vi "Apply Module Configuration Data.vi"(8 "Error In":errorcluster, 11 "Compiled.Settings":T1 {"Configuration Data"."Properties"."U64 Properties"."UInt64 Write" format="%.0x"; "Configuration Data"."Properties"."U32 Properties"."UInt32 Write" format="%.0x"; "Configuration Data"."Properties"."Double Properties"."Double Write" format="%_20g"}) -> (0 "Error Out":errorcluster, 2 "Device Session":refnum<k21>, 3 "SLSC Module Name":refnum<k21>)   [LabVIEW 2015, in "SLSC-12201 DIO Engine.lvlib"]
uses:
  SLSC-12201 DIO Engine.lvlib
  Shared/Compiled.Settings
  Shared/SLSC Dynamic Channel.ctl
  Shared/SLSC Dynamic Channel Type.ctl
  <vilib>/SLSC/Initialize Session with Devices.vi
  <vilib>/NI Veristand/Custom Device Tools/Custom Device Utility Library/Custom Device Utility Library.lvlib
  <vilib>/NI Veristand/Custom Device Tools/Custom Device Utility Library/RT Debug String Color Spec.ctl
  <vilib>/SLSC/SLSC.lvlib
  Shared/SLSC-12201 DIO Shared.lvlib
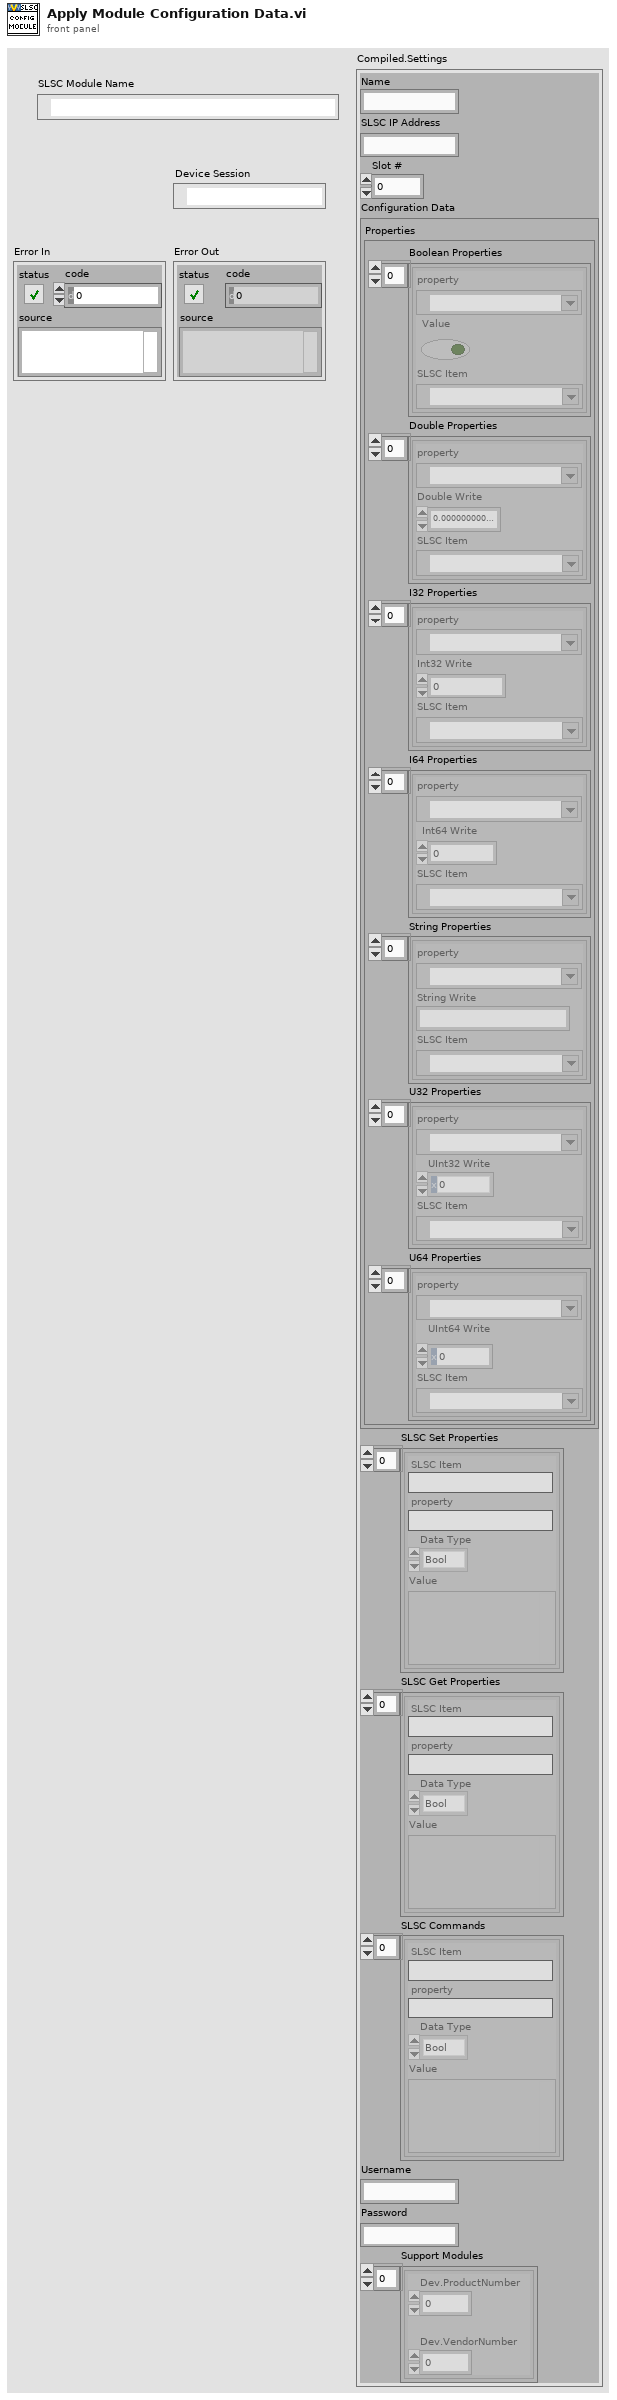
[diagram p1: front panel]
types:
  T1 = typedef "SLSC-12201 DIO Shared.lvlib/Compiled.Settings" = cluster{"Name":string, "SLSC IP Address":string, "Slot #":i32, "Configuration Data":cluster{"Properties":cluster{"Boolean Properties":cluster{"property":refnum<k21>, "Value":bool, "SLSC Item":refnum<k21>}[], "Double Properties":cluster{"property":refnum<k21>, "Double Write":dbl, "SLSC Item":refnum<k21>}[], "I32 Properties":cluster{"property":refnum<k21>, "Int32 Write":i32, "SLSC Item":refnum<k21>}[], "I64 Properties":cluster{"property":refnum<k21>, "Int64 Write":i64, "SLSC Item":refnum<k21>}[], "String Properties":cluster{"property":refnum<k21>, "String Write":string, "SLSC Item":refnum<k21>}[], "U32 Properties":cluster{"property":refnum<k21>, "UInt32 Write":u32, "SLSC Item":refnum<k21>}[], "U64 Properties":cluster{"property":refnum<k21>, "UInt64 Write":u64, "SLSC Item":refnum<k21>}[]}}, "SLSC Set Properties":T2[], "SLSC Get Properties":T2[], "SLSC Commands":T2[], "Username":string, "Password":string, "Support Modules":cluster{"Dev.ProductNumber":u32, "Dev.VendorNumber":u32}[]}
  T2 = typedef "SLSC-12201 DIO Shared.lvlib/SLSC Dynamic Channel.ctl" = cluster{"SLSC Item":string, "property":string, "Data Type":T3, "Value":variant}
  T3 = typedef "SLSC-12201 DIO Shared.lvlib/SLSC Dynamic Channel Type.ctl" = enum16{"Bool", "Double", "I32", "I64", "String", "U32", "U64", "EnumI32"}
  T4 = typedef "Custom Device Utility Library.lvlib/RT Debug String Color Spec.ctl" = u16
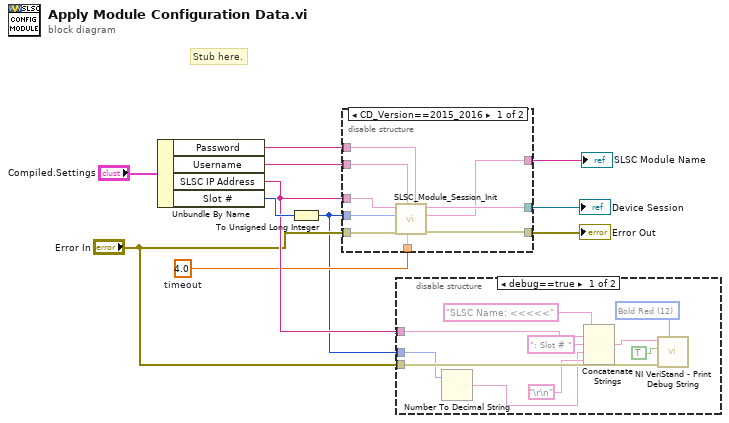
[diagram p0: block diagram]
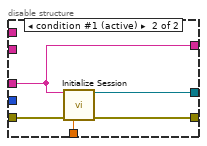
[diagram p3: hidden frame]
diagram:
  w7 = 4.0  # timeout
  # "Stub here."
  n1 = Unbundle By Name("Compiled.Settings") -> ("Password"=w5:string, "Username"=w6:string, "SLSC IP Address"=w9:string, "Slot #"=w10:i32)
  n2 = To Unsigned Long Integer(number=w10) -> (unsigned 32bit integer=w1:u32)
  n3 = disable-structure shown="CD_Version==2015_2016" {
    disable-tunnel: w1 -> [w20 _]
    disable-tunnel: w9 -> [w19 w23]
    disable-tunnel: "Error In" -> [w18 w22]
    disable-tunnel: w7 -> [w17 w25]
    disable-tunnel: w6 -> [w16 _]
    disable-tunnel: w5 -> [w15 _]
    disable-tunnel: [w14 w24] -> w4
    disable-tunnel: [w13 w23] -> w3
    disable-tunnel: [w12 w21] -> w2
    frame condition #0 {
      n4 = call "SLSC_Module_Session_Init.vi"("Password"=w15, "connect timeout (10 sec)"=w17, "Username"=w16, "Error In"=w18, "Slot #"=w20, "Chassis IP Address"=w19) -> ("Error Out"=w12:errorcluster, "SLSC Module Name"=w13:string, "Module Session Out"=w14:string)  [unwired: 2 in, 1 out]
    }
    frame condition #1 (active) {
      n5 = call-poly <vilib>:"Initialize Session.vi"("devices"=w23, "error in (no error)"=w22, "connect timeout (60 sec)"=w25) -> ("session out"=w24:refnum<k21>, "error out"=w21:errorcluster)  [unwired: 11 in]
    }
  }
  "Error Out" <- w2
  "Device Session" <- w4
  "SLSC Module Name" <- w3
  n6 = disable-structure shown="debug==true" {
    disable-tunnel: w9 -> [w35 _]
    disable-tunnel: "Error In" -> [w34 _]
    disable-tunnel: w1 -> [w27 _]
    frame condition #0 {
      w30 = T4 12 items=["Plain White"=7, "Bold White"=15, "Bold Blue"=9, "Bold Green"=10, "Bold Red"=12] ("Attribute")
      n7 = Number To Decimal String(number=w27) -> (decimal integer string=w26:string)  [unwired: 1 in]
      n8 = Concatenate Strings("SLSC Name: <<<<<" ("string"), w35, ": Slot # " ("string"), w26, "\r\n") -> (w33:string)
      n9 = call <vilib>:"NI VeriStand - Print Debug String.vi"("Attribute"=w30, "error in (no error)"=w34, "Add to log file? (T)"=TRUE, "Message"=w33) -> ()  [unwired: 7 in, 1 out]
    }
    frame condition #1 (active) {
    }
  }
